vi "Calculate 1D scan positions.vi"(2 "Scan direction":u16(ring) items=["Left & right (- & +)", "To the left (-)", "To the right (+)"], 3 "Start position":dbl format="%.6f", 6 "Range":dbl format="%.2f", 7 "Step size":dbl format="%.2f") -> (14 "1D position array":dbl[](array[numeric]) format="%.6f", 15 "Minimum position":dbl format="%.6f", 16 "Maximum position":dbl format="%.6f", 17 "No. of steps":i32, 18 "1D intensity array":dbl[](array[numeric]) format="%.6f")   [LabVIEW 2026]
doc: "Calculates 1D scan positions according to Scan direction, Start position, Range and Step size and returns Minimum position, Maximum position, No. of steps and initialized 1D position array and 1D intensity array. Scan direction can be \n- Left & right (- & +) meaning that the scan starts at (Start position - ½ Range) and stops at (Start position + ½ Range), \n- To the left (-) meaning that scan starts (Start position - Range) and stops at Start position, or \n- To the right (+) meaning that scan starts at Start position and stops at (Start position + Range)."
panel:
  # "Calculates 1D scan positions and initializes intensity array."
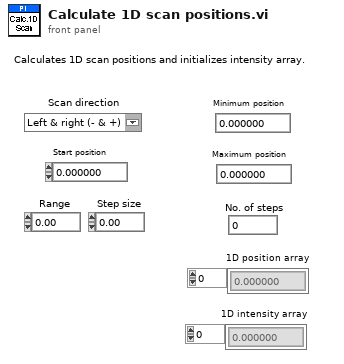
[diagram p1: front panel]
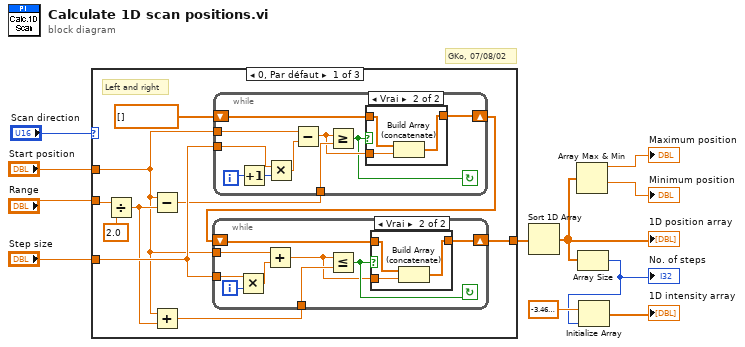
[diagram p0: block diagram]
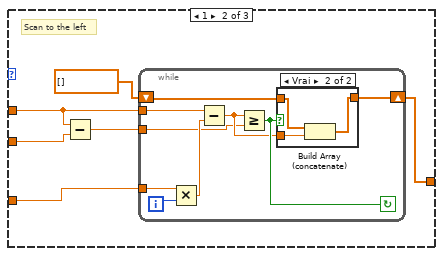
[diagram p4: hidden frame]
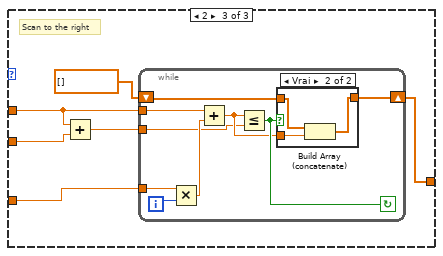
[diagram p6: hidden frame]
diagram:
  # "GKo, 07/08/02"
  n1 = case shown="0, Par défaut" "Scan direction" {
    tunnel: "Range" -> [w21 w52 w71]
    tunnel: "Start position" -> [w16 w53 w72]
    tunnel: "Step size" -> [w18 w54 w73]
    tunnel: [w12 w49 w68] -> w2
    frame 0, Default {
      # "Left and right"
      n2 = Divide(x=w21, y=2.0) -> (x/y=w17:dbl)
      n3 = Subtract(x=w16, y=w17) -> (x-y=w15:dbl)
      n4 = Add(x=w16, y=w17) -> (x+y=w19:dbl)
      n5 = while {
        shift-left: dbl[] [] -> [w38]
        shift-right: [w36] -> w13
        tunnel: w15 -> [w39]
        tunnel: w18 -> [w41]
        tunnel: w16 -> [w43]
        i -> [w44]
        stop <- w35 continue-if-true
        n6 = Increment(x=w44) -> (x+1=w42:i32)
        n7 = Multiply(x=w41, y=w42) -> (x*y=w40:dbl)
        n8 = Subtract(x=w43, y=w40) -> (x-y=w37:dbl)
        n9 = Greater Or Equal?(x=w37, y=w39) -> (x >= y?=w35:bool)
        n10 = case shown="Vrai" w35 {
          tunnel: [w45 w48] -> w36
          tunnel: w38 -> [w45 w47]
          tunnel: w37 -> [_ w46]
          frame False {
          }
          frame True {
            n11 = Build Array (concatenate)(w47, w46) -> (w48:dbl[])
          }
        }
      }
      n12 = while {
        tunnel: w19 -> [w24]
        shift-left: w13 -> [w25]
        shift-right: [w26] -> w12
        tunnel: w16 -> [w28]
        tunnel: w18 -> [w29]
        i -> [w30]
        stop <- w23 continue-if-true
        n13 = Multiply(x=w29, y=w30) -> (x*y=w27:dbl)
        n14 = Add(x=w28, y=w27) -> (x+y=w22:dbl)
        n15 = Less Or Equal?(x=w22, y=w24) -> (x <= y?=w23:bool)
        n16 = case shown="Vrai" w23 {
          tunnel: [w31 w34] -> w26
          tunnel: w25 -> [w31 w33]
          tunnel: w22 -> [_ w32]
          frame False {
          }
          frame True {
            n17 = Build Array (concatenate)(w33, w32) -> (w34:dbl[])
          }
        }
      }
    }
    frame 1 {
      # "Scan to the left"
      n18 = Subtract(x=w53, y=w52) -> (x-y=w51:dbl)
      n19 = while {
        tunnel: w51 -> [w55]
        shift-left: dbl[] [] -> [w59]
        shift-right: [w58] -> w49
        tunnel: w54 -> [w61]
        tunnel: w53 -> [w63]
        i -> [w62]
        stop <- w57 continue-if-true
        n20 = Multiply(x=w61, y=w62) -> (x*y=w60:dbl)
        n21 = Subtract(x=w63, y=w60) -> (x-y=w56:dbl)
        n22 = Greater Or Equal?(x=w56, y=w55) -> (x >= y?=w57:bool)
        n23 = case shown="Vrai" w57 {
          tunnel: [w64 w67] -> w58
          tunnel: w59 -> [w64 w66]
          tunnel: w56 -> [_ w65]
          frame False {
          }
          frame True {
            n24 = Build Array (concatenate)(w66, w65) -> (w67:dbl[])
          }
        }
      }
    }
    frame 2 {
      # "Scan to the right"
      n25 = Add(x=w72, y=w71) -> (x+y=w70:dbl)
      n26 = while {
        tunnel: w70 -> [w74]
        shift-left: dbl[] [] -> [w78]
        shift-right: [w77] -> w68
        tunnel: w73 -> [w80]
        tunnel: w72 -> [w82]
        i -> [w81]
        stop <- w76 continue-if-true
        n27 = Multiply(x=w80, y=w81) -> (x*y=w79:dbl)
        n28 = Add(x=w82, y=w79) -> (x+y=w75:dbl)
        n29 = Less Or Equal?(x=w75, y=w74) -> (x <= y?=w76:bool)
        n30 = case shown="Vrai" w76 {
          tunnel: [w83 w86] -> w77
          tunnel: w78 -> [w83 w85]
          tunnel: w75 -> [_ w84]
          frame False {
          }
          frame True {
            n31 = Build Array (concatenate)(w85, w84) -> (w86:dbl[])
          }
        }
      }
    }
  }
  n32 = Sort 1D Array(array=w2) -> (sorted array=w4:dbl[])
  "1D position array" <- w4
  n33 = Array Max & Min(array=w4) -> (max value=→"Maximum position":dbl, min value=→"Minimum position":dbl)  [unwired: 2 out]
  n34 = Array Size(array=w4) -> (size(s)=w1:i32)
  "No. of steps" <- w1
  n35 = Initialize Array(-3.469446951953614e-18 ("Element Data"), w1) -> (→"1D intensity array":dbl[])
